vi "2401 Scratch.vi"(10 "Current Level (A)":dbl) -> (1 "Resistance":dbl format="%#_6e", 2 "Current":dbl format="%#_6e", 3 "Voltage":dbl format="%_6e")   [LabVIEW 2009]
panel:
  out "number 4":dbl format="%#_6e"
  out "number5":dbl format="%#_6e"
  out "read buffer":string
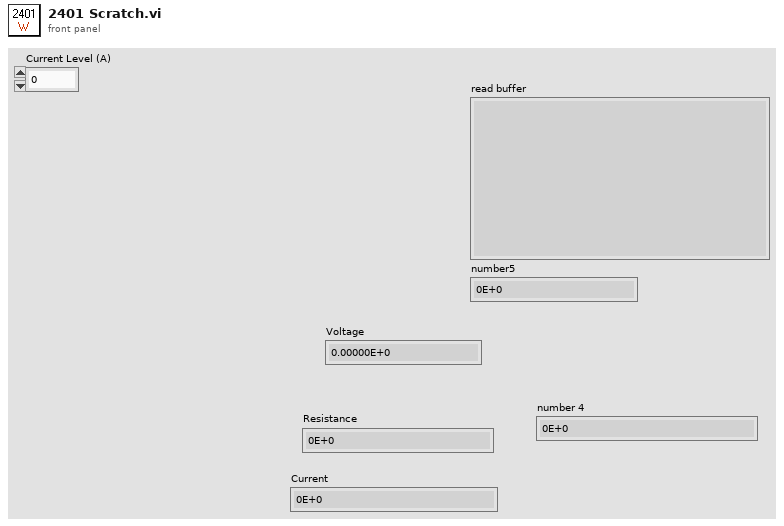
[diagram p1: front panel]
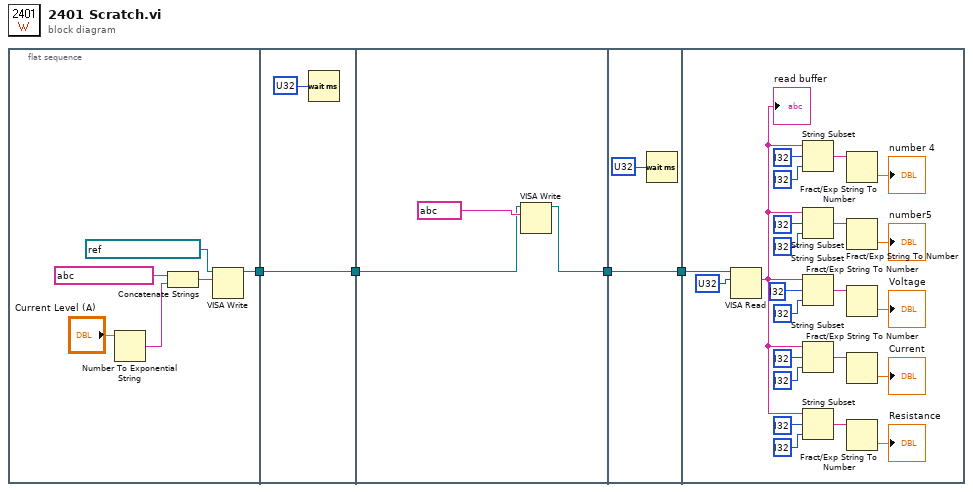
[diagram p0: block diagram]
diagram:
  n1 = flat-sequence {
    tunnel: [w9] -> w4
    tunnel: w4 -> [w12]
    tunnel: [w12] -> w3
    tunnel: w3 -> [w14]
    tunnel: [w13] -> w2
    tunnel: w2 -> [w17]
    tunnel: [w17] -> w1
    tunnel: w1 -> [w40]
    frame #0 {
      n2 = Number To Exponential String(number="Current Level (A)") -> (E-format string=w6:string)  [unwired: 3 in]
      n3 = Concatenate Strings(string ? ("write buffer"), w6) -> (w7:string)
      n4 = VISA Write(VISA resource name=refnum<visa-resource-name> ?, write buffer=w7) -> (VISA resource name out=w9:refnum<visa-resource-name>)  [unwired: 1 in, 2 out]
    }
    frame #1 {
      n5 = Wait (ms)(milliseconds to wait=u32 ?) -> ()  [unwired: 1 out]
    }
    frame #2 {
      n6 = VISA Write(VISA resource name=w14, write buffer=string ?) -> (VISA resource name out=w13:refnum<visa-resource-name>)  [unwired: 1 in, 2 out]
    }
    frame #3 {
      n7 = Wait (ms)(milliseconds to wait=u32 ?) -> ()  [unwired: 1 out]
    }
    frame #4 {
      n8 = VISA Read(VISA resource name=w40, byte count=u32 ?) -> (read buffer=w18:string)  [unwired: 1 in, 3 out]
      "read buffer" <- w18
      n9 = String Subset(string=w18, offset (0)=i32 ?, length (rest)=i32 ? ("length (rest)")) -> (substring=w20:string)
      n10 = String Subset(string=w18, offset (0)=i32 ?, length (rest)=i32 ? ("length (rest)")) -> (substring=w36:string)
      n11 = String Subset(string=w18, offset (0)=i32 ?, length (rest)=i32 ? ("length (rest)")) -> (substring=w32:string)
      n12 = String Subset(string=w18, offset (0)=i32 ?, length (rest)=i32 ? ("length (rest)")) -> (substring=w28:string)
      n13 = String Subset(string=w18, offset (0)=i32 ?, length (rest)=i32 ? ("length (rest)")) -> (substring=w24:string)
      n14 = Fract/Exp String To Number(string=w20) -> (number=→"number 4":dbl)  [unwired: 3 in, 1 out]
      n15 = Fract/Exp String To Number(string=w36) -> (number=→"number5":dbl)  [unwired: 3 in, 1 out]
      n16 = Fract/Exp String To Number(string=w32) -> (number=→"Voltage":dbl)  [unwired: 3 in, 1 out]
      n17 = Fract/Exp String To Number(string=w28) -> (number=→"Current":dbl)  [unwired: 3 in, 1 out]
      n18 = Fract/Exp String To Number(string=w24) -> (number=→"Resistance":dbl)  [unwired: 3 in, 1 out]
    }
  }
